vi "1.5子程序.vi"(1 "value2":dbl, 2 "value1":dbl) -> (0 "max_value":dbl)   [LabVIEW 2016]
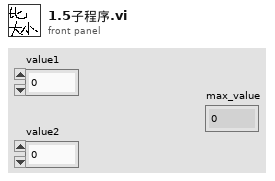
[diagram p1: front panel]
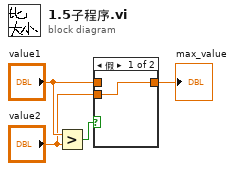
[diagram p0: block diagram]
diagram:
  n1 = Greater?(x="value1", y="value2") -> (0:w4:bool)
  n2 = case shown="假" w4 {
    tunnel: "value1" -> [_ w6]
    tunnel: "value2" -> [w5 _]
    tunnel: [w5 w6] -> w1
    frame False {
    }
    frame True {
    }
  }
  "max_value" <- w1
